vi "Fdx Close Session.vi"   [LabVIEW 2020, in "AIM664LV.lvlib"]
uses:
  AIM664LV.lvlib
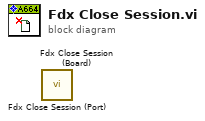
[diagram p0: block diagram]
diagram:
  n1 = call "Fdx Close Session (Port).vi"() -> ()  [unwired: 11 in, 1 out]
  n2 = call "Fdx Close Session (Board).vi"() -> ()  [unwired: 11 in, 1 out]
